vi "set file meta.vi"(8 "error in (no error)":errorcluster, 11 "5785_3.2GHz_one channel in":refnum<class "5785_3.2GHz_one channel.lvclass">) -> (0 "error out":errorcluster, 3 "5785_3.2GHz_one channel out":refnum<class "5785_3.2GHz_one channel.lvclass">)   [LabVIEW 2021, in "5785_3.2GHz_one channel.lvclass"]
uses:
  5785_3.2GHz_one channel.lvclass
  pulse_tx_vis/CTL/device_mode.ctl
  5785_3.2GHz_one channel.lvclass/5785_3.2GHz_one channel.ctl
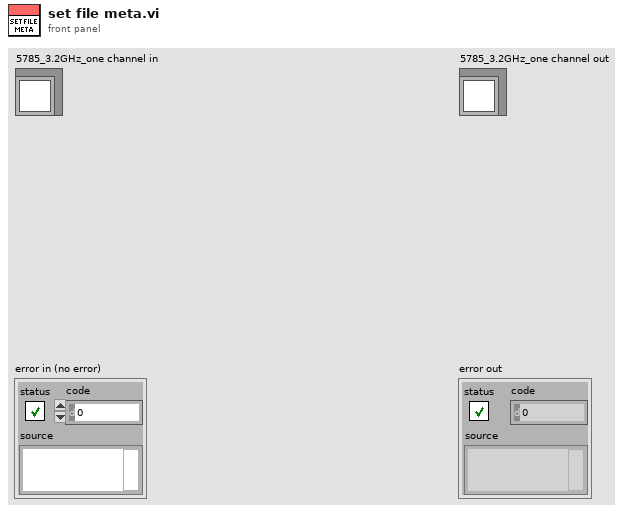
[diagram p1: front panel]
types:
  T1 = typedef "device_mode.ctl" = enum16{"USRP - 180MHz", "5785 - 2*180MHz", "5785 - 3.2GHz", "P2P - VST", "5785 2*1.6GHz"}
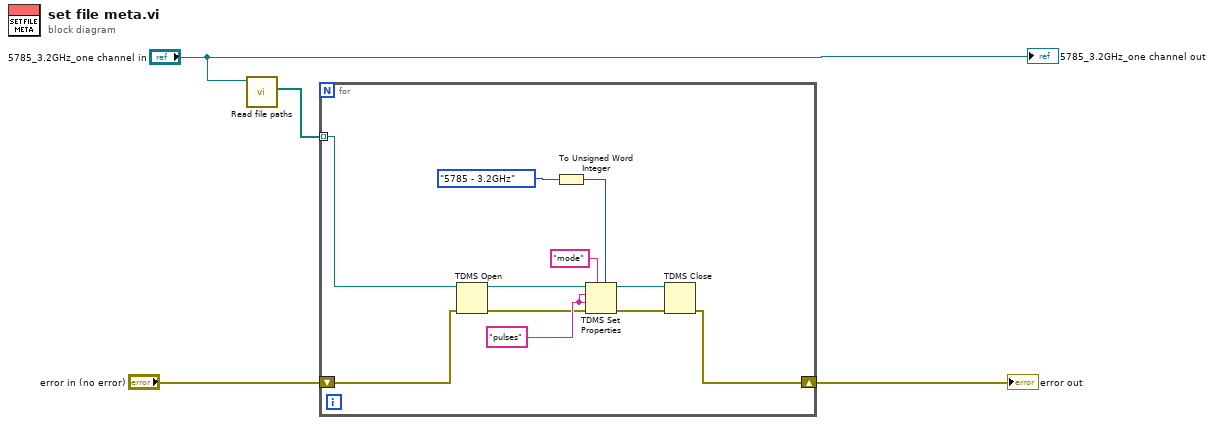
[diagram p0: block diagram]
diagram:
  n1 = call-dynamic "Read file paths.vi"("device_type in"="5785_3.2GHz_one channel in") -> ("file paths"=w4:path[])  [unwired: 8 in, 2 out]
  n2 = for {
    tunnel: w4 -> [w13] mode=indexing
    shift-right: [w5] -> w2
    shift-left: "error in (no error)" -> [w6]
    w15 = "pulses" ("channel name")
    n3 = TDMS Open(8:w6, 11:w13) -> (0:w10:errorcluster, 3:w14:refnum<k34>)  [unwired: 5 in]
    n4 = To Unsigned Word Integer(number=device_mode."5785 - 3.2GHz" ("Mode")) -> (unsigned 16bit integer=w7:u16)
    n5 = TDMS Set Properties(5:w7, 7:"mode", 8:w10, 9:w15, 10:w15, 11:w14) -> (0:w11:errorcluster, 3:w12:refnum<k34>)  [unwired: 2 out]
    n6 = TDMS Close(8:w11, 11:w12) -> (0:w5:errorcluster)  [unwired: 1 out]
  }
  "error out" <- w2
  "5785_3.2GHz_one channel out" <- "5785_3.2GHz_one channel in"
